vi "SSC Digital Get Fail Count.vi"(0 "Digital SSC in":T1[](array[typedef]), 11 "error in":errorcluster) -> (4 "Digital SSC out":T1[](array[typedef]), 6 "Per-Instrument Failure Counts":i64[][](array[numeric]), 15 "error out":errorcluster)   [LabVIEW 2019]
doc: "Returns the comparison fail count for the specified pin(s) and pin group(s)."
uses:
  SSC Digital.ctl
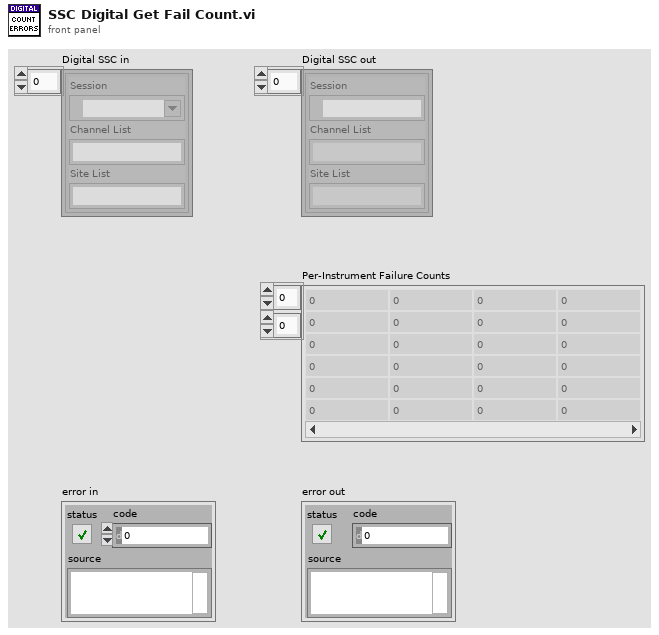
[diagram p1: front panel]
types:
  T1 = typedef "SSC Digital.ctl" = cluster{"Session":refnum<k15>, "Channel List":string, "Site List":string}
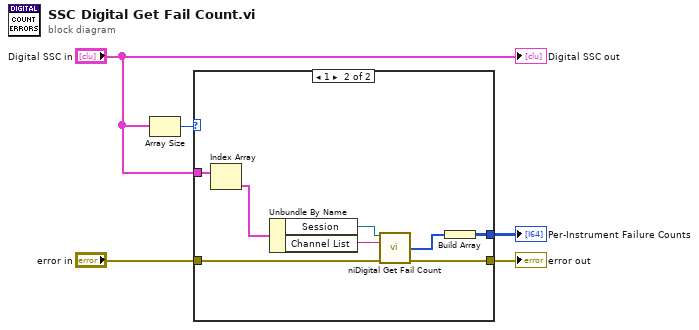
[diagram p0: block diagram]
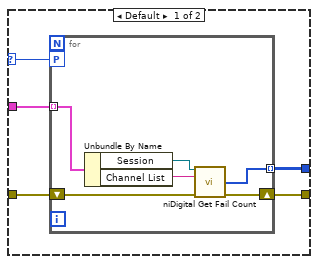
[diagram p2: hidden frame]
diagram:
  n1 = Array Size(array="Digital SSC in") -> (size(s)=w2:i32)
  n2 = case shown="1" w2 {
    selector: w2 -> [w7 _]
    tunnel: "error in" -> [w10 w24]
    tunnel: [w9 w17] -> w4
    tunnel: [w8 w22] -> w3
    tunnel: "Digital SSC in" -> [w6 w21]
    frame Default {
      n3 = for {
        tunnel: [w14] -> w9 mode=indexing
        workers-P: w7 -> [_]
        tunnel: w6 -> [w13] mode=indexing
        shift-right: [w15] -> w8
        shift-left: w10 -> [w16]
        n4 = Unbundle By Name(w13) -> ("Session"=w12:refnum<k15>, "Channel List"=w11:string)
        n5 = call <instrlib>:"niDigital Get Fail Count.vi"("instrument handle"=w12, "channel list"=w11, "error in"=w16) -> ("failure count"=w14:i64[], "error out"=w15:errorcluster)  [unwired: 10 in, 1 out]
      }
    }
    frame 1 {
      n6 = Index Array(array=w21) -> (element=w18:T1)  [unwired: 1 in]
      n7 = Unbundle By Name(w18) -> ("Session"=w20:refnum<k15>, "Channel List"=w19:string)
      n8 = call <instrlib>:"niDigital Get Fail Count.vi"("instrument handle"=w20, "channel list"=w19, "error in"=w24) -> ("failure count"=w23:i64[], "error out"=w22:errorcluster)  [unwired: 10 in, 1 out]
      n9 = Build Array(w23) -> (w17:i64[][])
    }
  }
  "error out" <- w3
  "Per-Instrument Failure Counts" <- w4
  "Digital SSC out" <- "Digital SSC in"
